vi "check for zeros.vi"(10 "number of zeros numérique":i32=-1, 11 "Array":u16[](array[numeric])) -> (3 "Yes/No":bool)   [LabVIEW 2020, in "VIS-NIR.lvclass"]
uses:
  Classes/Detector/VIS-IR/VIS-NIR.lvclass
  globalVarII.vi
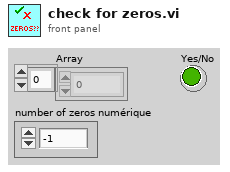
[diagram p1: front panel]
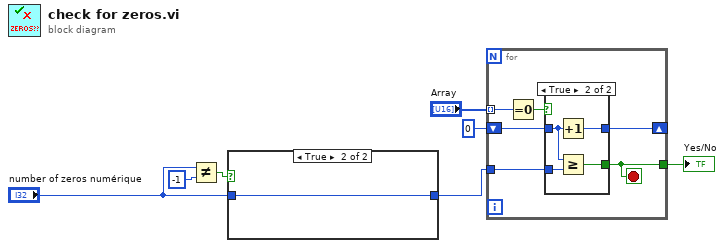
[diagram p0: block diagram]
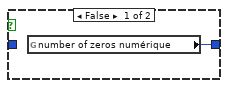
[diagram p2: hidden frame]
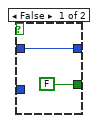
[diagram p3: hidden frame]
diagram:
  n1 = Not Equal?(x="number of zeros numérique", y=-1) -> (x != y?=w3:bool)
  n2 = case shown="True" w3 {
    tunnel: [w8 w9] -> w1
    tunnel: "number of zeros numérique" -> [_ w9]
    frame False {
      n3 = global read "globalVarII.vi" "number of zeros numérique"() -> (w8:i32)
    }
    frame True {
    }
  }
  n4 = for {
    tunnel: "Array" -> [w15] mode=indexing
    shift-right: [w12] -> _
    shift-left: 0 -> [w14]
    tunnel: [w11] -> w5
    tunnel: w1 -> [w10]
    stop <- w11 stop-if-true
    n5 = Equal To 0?(x=w15) -> (x = 0?=w13:bool)
    n6 = case shown="True" w13 {
      tunnel: w14 -> [w17 w20]
      tunnel: [w17 w21] -> w12
      tunnel: w10 -> [_ w19]
      tunnel: [FALSE w18] -> w11
      frame False {
      }
      frame True {
        n7 = Increment(x=w20) -> (x+1=w21:i32)
        n8 = Greater Or Equal?(x=w20, y=w19) -> (x >= y?=w18:bool)
      }
    }
  }
  "Yes/No" <- w5
